vi "mupLib EvalBulk example.vi"() -> ()   [LabVIEW 2015]
uses:
  mupLib/mupLibPath.vi
  mupLib/mupCheckError.vi
  <vilib>/Utility/error.llb/Error Cluster From Error Code.vi
  mupLib/mupLib.lvlib
panel:
  out "Results":dbl[][](array[numeric])
  out "error out":errorcluster
  in  "c":dbl=3.0
  in  "Expression":string="a*x^2+b*x+c"
  in  "b":dbl=2.0
  in  "a":dbl=1.0
  # "Constants"
  # "x Values"
  # "Results"
  # "This example demonstrates bulk mode evaluation using mupLib.\n\n- Enter an expression containing constants a, b, c, and variable x.\n- Enter values for constants a, b, c.\n- Hit run to evaluate the expression for x values of 0-999"
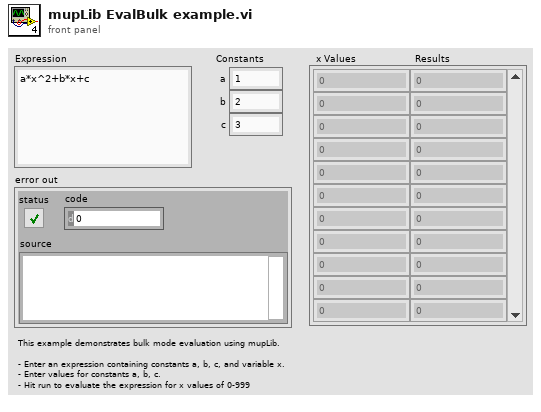
[diagram p1: front panel]
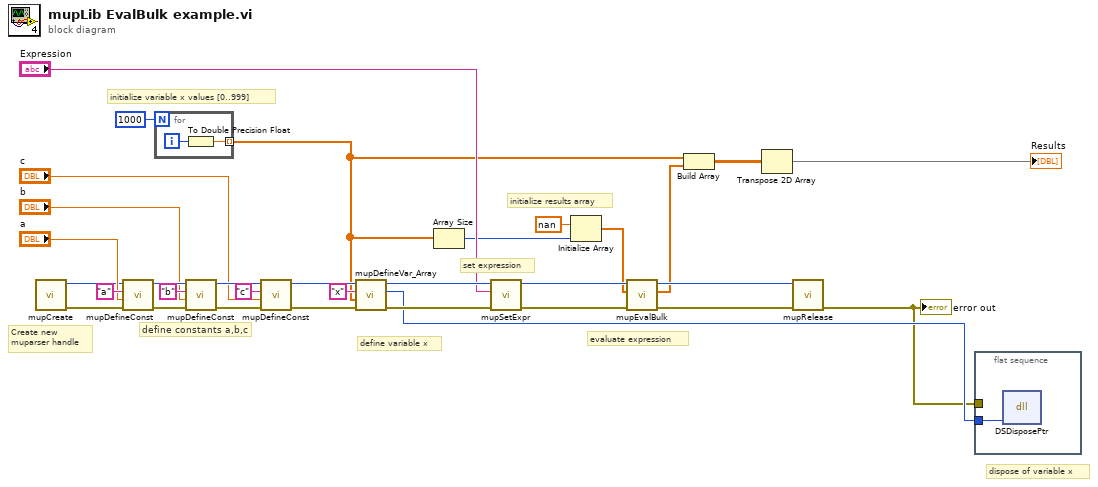
[diagram p0: block diagram]
diagram:
  # "initialize variable x values [0..999]"
  # "dispose of variable x"
  # "evaluate expression"
  # "initialize results array"
  # "set expression"
  # "define variable x"
  # "define constants a,b,c"
  # "Create new\nmuparser handle"
  n1 = call "mupCreate.vi"() -> ("error out"=w32:errorcluster, "hParser out"=w15:u64)  [unwired: 10 in]
  n2 = call "mupDefineConst.vi"("error in (no error)"=w32, "Value"="a", "constName"="a", "hParser in"=w15) -> ("error out"=w27:errorcluster, "hParser out"=w28:u64)  [unwired: 6 in]
  n3 = for {
    N: 1000 -> [_]
    tunnel: [w33] -> w4 mode=indexing
    i -> [w34]
    n4 = To Double Precision Float(number=w34) -> (double precision float=w33:dbl)
  }
  n5 = call "mupDefineConst.vi"("error in (no error)"=w27, "Value"="b", "constName"="b", "hParser in"=w28) -> ("error out"=w19:errorcluster, "hParser out"=w20:u64)  [unwired: 6 in]
  n6 = call "mupDefineConst.vi"("error in (no error)"=w19, "Value"="c", "constName"="c", "hParser in"=w20) -> ("error out"=w17:errorcluster, "hParser out"=w16:u64)  [unwired: 6 in]
  n7 = call "mupDefineVar_Array.vi"("error in (no error)"=w17, "initValue"=w4, "varName"="x", "hParser in"=w16) -> ("error out"=w22:errorcluster, "varAddr"=w14:u64, "hParser out"=w24:u64)  [unwired: 5 in]
  n8 = Array Size(array=w4) -> (size(s)=w7:i32)
  n9 = call "mupSetExpr.vi"("error in (no error)"=w22, "szExpr"="Expression", "muPar in"=w24) -> ("error out"=w12:errorcluster, "muPar out"=w13:u64)  [unwired: 7 in]
  n10 = Initialize Array(nan ("element"), w7) -> (w6:dbl[])
  n11 = call "mupEvalBulk.vi"("error in (no error)"=w12, "a_res"=w6, "hParser in"=w13) -> ("error out"=w10:errorcluster, "results"=w3:dbl[], "hParser out"=w11:u64)  [unwired: 6 in]
  n12 = Build Array(w4, w3) -> (w2:dbl[][])
  n13 = Transpose 2D Array(2D array=w2) -> (transposed array=→"Results":dbl[][])
  n14 = call "mupRelease.vi"("error in (no error)"=w10, "hParser in"=w11) -> ("error out"=w9:errorcluster)  [unwired: 9 in]
  "error out" <- w9
  n15 = flat-sequence {
    tunnel: w14 -> [w35]
    tunnel: w9 -> [_]
    frame #0 {
      n16 = dll-call lib="LabVIEW" fn="DSDisposePtr"("ptr"=w35) -> ()  [unwired: 5 in, 2 out]
    }
  }
